vi "Convert String to Byte Array.vi"(11 "rawData in":string[](array[string])) -> (3 "Array out":u8[][](array[numeric]))   [LabVIEW 2020]
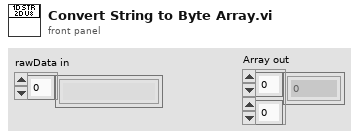
[diagram p1: front panel]
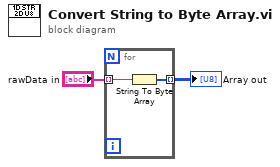
[diagram p0: block diagram]
diagram:
  n1 = for {
    tunnel: "rawData in" -> [w4] mode=indexing
    tunnel: [w3] -> w1 mode=indexing
    n2 = String To Byte Array(string=w4) -> (unsigned byte array=w3:u8[])
  }
  "Array out" <- w1
